vi "Get gRPC Method Name.vi"(8 "error in (no error)":errorcluster, 11 "Method ref in":u64) -> (0 "error out":errorcluster, 2 "Method Name":string, 3 "Method ref out":u64)   [LabVIEW 2019, in "gRPC Template Creation Utility.lvlib"]
uses:
  gRPC Template Creation Utility.lvlib
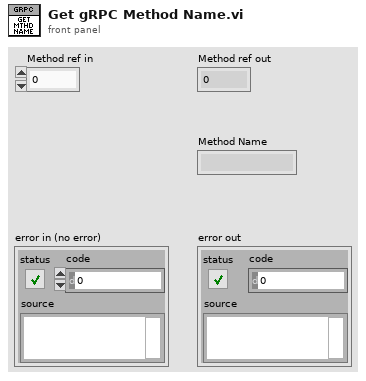
[diagram p1: front panel]
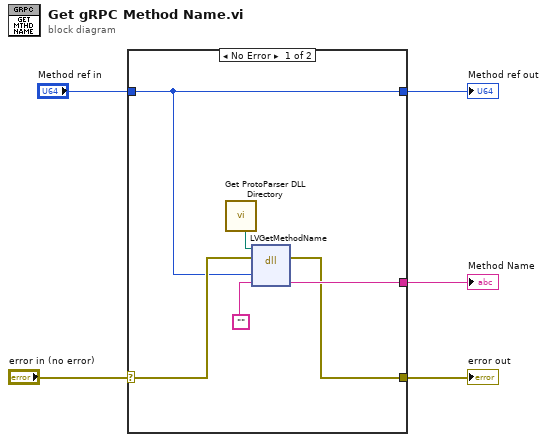
[diagram p0: block diagram]
diagram:
  n1 = case shown="No Error" "error in (no error)" {
    selector: "error in (no error)" -> [w8 w13]
    tunnel: "Method ref in" -> [w7 w12]
    tunnel: [w11 _] -> w4
    tunnel: [w7 w12] -> w2
    tunnel: [w6 w13] -> w1
    frame No Error {
      n2 = call "Get ProtoParser DLL Directory.vi"() -> ("Proto Parser Directory"=w9:path)
      n3 = dll-call lib="C:/Users/XEnderMD/Desktop/LV gRPC/labview source/gRPC Scripting Tools/Proto Parser API/dll/labview_grpc_generator.dll" fn="LVGetMethodName"(path in=w9, error in=w8, "method"=w7, "methodName"="") -> (error out=w6:errorcluster, "methodName"=w11:string)  [unwired: 3 in, 1 out]
    }
    frame Error {
    }
  }
  "Method Name" <- w4
  "Method ref out" <- w2
  "error out" <- w1
